vi "Vision Processing.vi"(8 "error in (no error)":errorcluster, 11 "Image Size":T2=enum."320x240") -> ()   [LabVIEW 2015]
uses:
  <vilib>/Rock Robotics/WPI/Camera/WPI_CameraImageSize.ctl
  SubSystems/Vision Support Code/Camera Types.ctl
  <vilib>/Rock Robotics/WPI/Camera/WPI_CameraFrameRate.ctl
  <vilib>/Rock Robotics/WPI/Camera/WPI_CameraWhite Balance Values.ctl
  <vilib>/Rock Robotics/WPI/Camera/WPI_CameraExposure Values.ctl
  Robot Global Data.vi
  <vilib>/vision/NI_Vision_Development_Module.lvlib
panel:
  in  "Frame Rate (fps)":T1=30 min=1 max=30
  in  "Image Size 2":T2=enum."320x240"
  in  "Goal Width":dbl=20.0
  in  "Center Right":dbl=170.0
  in  "Center Left":dbl=150.0
  in  "Maximum Shooting Distance":dbl
  in  "Distance Method":u16(ring)=2 items=["Default", "Center Calculations", "Hybrid", "Ratios"]
  in  "Camera Distance\nfrom Ground (in)":dbl
  out "More Detection":T3(array[cluster])
  in  "Mask Color":i32=1
  in  "Camera Type":T4=enum."MS HD3000 640x480"
  out "ms to process":u32
  in  "LED Color":T5={"Hue"={91.12518353230051, 179.40124989546868}, "Sat"={197.32142857142858, 255.0}, "Val"={182.14285714285714, 255.0}} {"Hue" scale=0.0..255.0 scale format="%#_3g"}
  out "Qualified Particles":i32
  in  "Aspect Fudge Factor":dbl=1.0
  in  "Min Score Threshold":i32=75
  out "Masked":T6(plugin-control)
  out "Original Image":T6(plugin-control)
  out "Sorted Particle Scores":T7(array[cluster]) {"Moment Factor" format="%#_3g"; "Aspect Ratio" format="%#_3g"; "Area to CH" format="%#_3g"; "X" format="%#_3g"; "Y" format="%#_3g"}
  out "Highest Avg Score":dbl
  out "Detected Targets":T8(array[cluster]) {"Normalized Rect"."Numeric 5" format="%#_2g"; "Normalized Rect"."Numeric 3" format="%#_2g"; "Normalized Rect"."Numeric 2" format="%#_2g"; "Normalized Rect"."Numeric" format="%#_2g"}
  out "fps":dbl
  # "Density Profile"
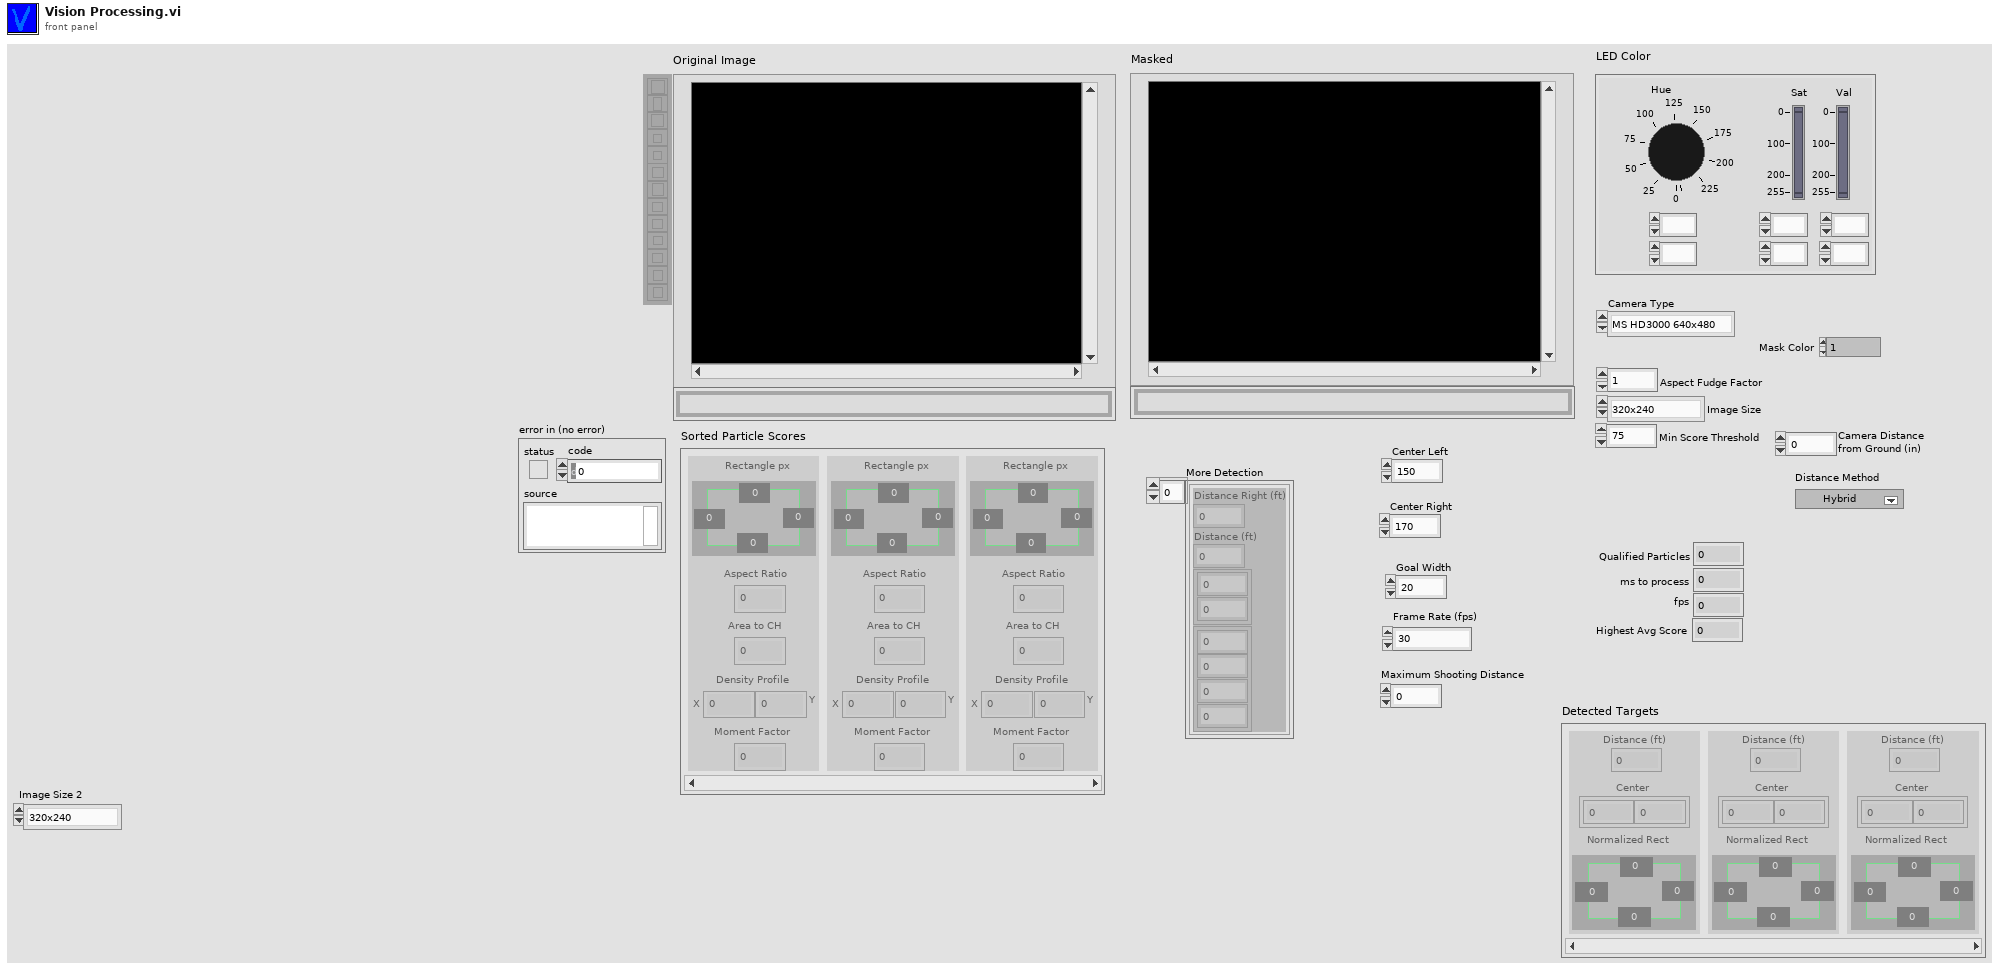
[diagram p1: front panel]
types:
  T1 = typedef "WPI_CameraFrameRate.ctl" = u32
  T2 = typedef "WPI_CameraImageSize.ctl" = enum16{"640x480", "320x240", "160x120", "Custom"}
  T3 = cluster{"Distance Right (ft)":dbl, "Distance (ft)":dbl, cluster{dbl, dbl}, cluster{dbl, dbl, dbl, dbl}}[]
  T4 = typedef "Camera Types.ctl" = enum16{"206", "1011", "1013", "MS HD3000 square", "MS HD3000 640x480"}
  T5 = cluster{"Hue":cluster{dbl, dbl}, "Sat":cluster{dbl, dbl}, "Val":cluster{dbl, dbl}}
  T6 = typedef "IMAQ Image.ctl" = refnum<image>
  T7 = cluster{"Rectangle px":cluster{"Numeric":dbl, "Numeric 2":dbl, "Numeric 3":dbl, "Numeric 5":dbl}, "Aspect Ratio":dbl, "Area to CH":dbl, "X":dbl, "Y":dbl, "Moment Factor":dbl}[]
  T8 = cluster{"Distance (ft)":dbl, "Center":cluster{dbl, dbl}, "Normalized Rect":cluster{"Numeric":dbl, "Numeric 2":dbl, "Numeric 3":dbl, "Numeric 5":dbl}}[]
  T9 = typedef "WPI_CameraExposure Values.ctl" = enum16{"Auto", "Flicker-free 50 Hz", "Flicker-free 60 Hz", "Hold current", "Custom"}
  T10 = typedef "WPI_CameraWhite Balance Values.ctl" = enum16{"Auto", "Fixed indoor", "Fixed outdoor 1", "Fixed outdoor 2", "Fixed fluorescent 1", "Fixed fluorescent 2", "Hold current", "Custom"}
  T11 = typedef "Image Type" = u32
  T12 = typedef "Particle Parameters" = i32
  T13 = typedef "WPI_CameraDevRef.ctl" = cluster{"Camera Address":string, "CameraStatus":errorcluster}
  T14 = cluster{"Bounding box":cluster{"left":dbl, "top":dbl, "right":dbl, "bottom":dbl}, "Aspect Ratio":dbl, "Area to CH":dbl, "X Mask":dbl, "Y Mask":dbl, "Moment":dbl}[]
  T15 = cluster{"Numeric":dbl, "Numeric":dbl, dbl, dbl, "Numeric":dbl, "Numeric":dbl}[]
  T16 = cluster{"Rectangle":cluster{"Numeric":dbl, "Numeric 2":dbl, "Numeric 3":dbl, "Numeric 5":dbl}, "L":dbl, "Area to CH":dbl, "X":dbl, "Y":dbl, "Moment Factor":dbl}[]
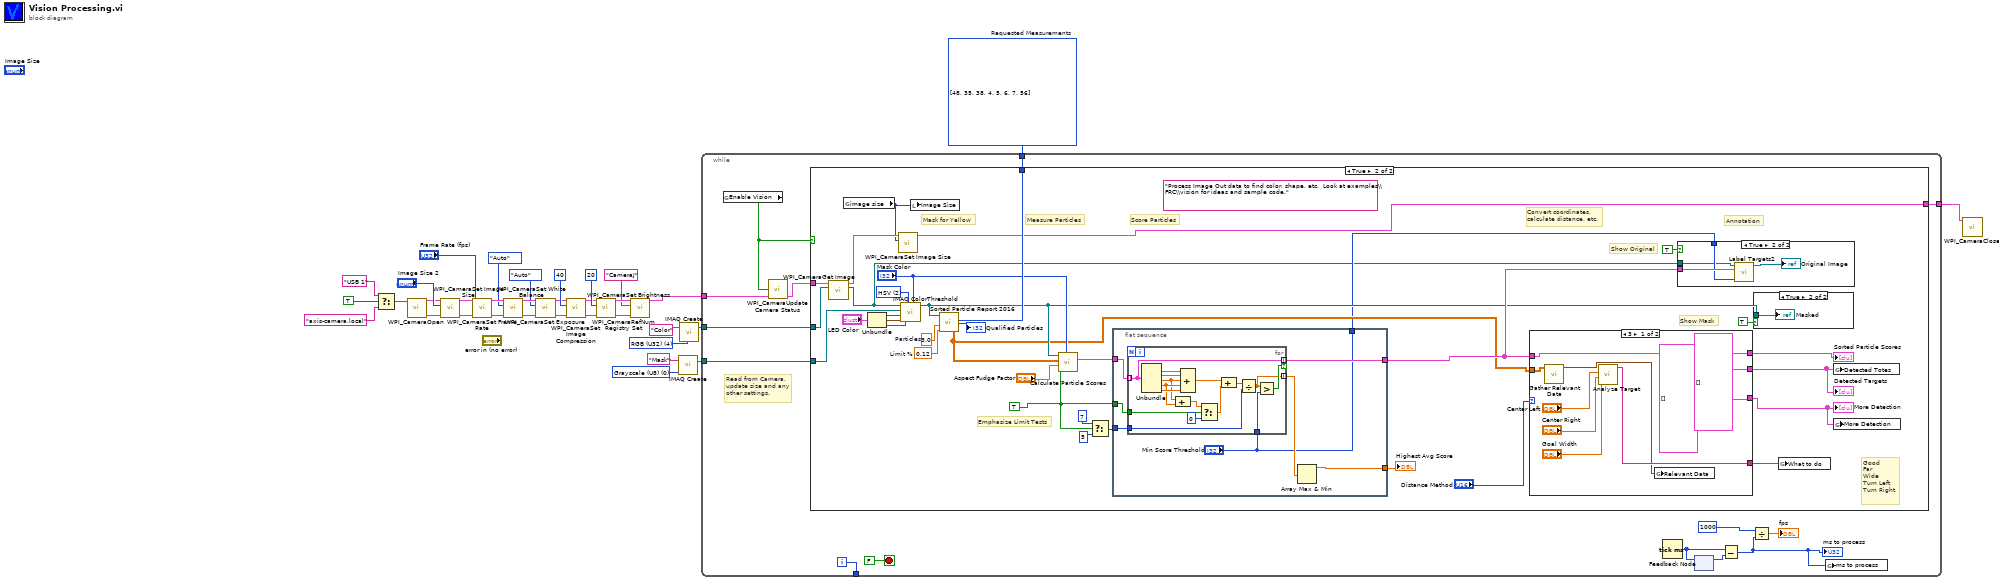
[diagram p0: block diagram]
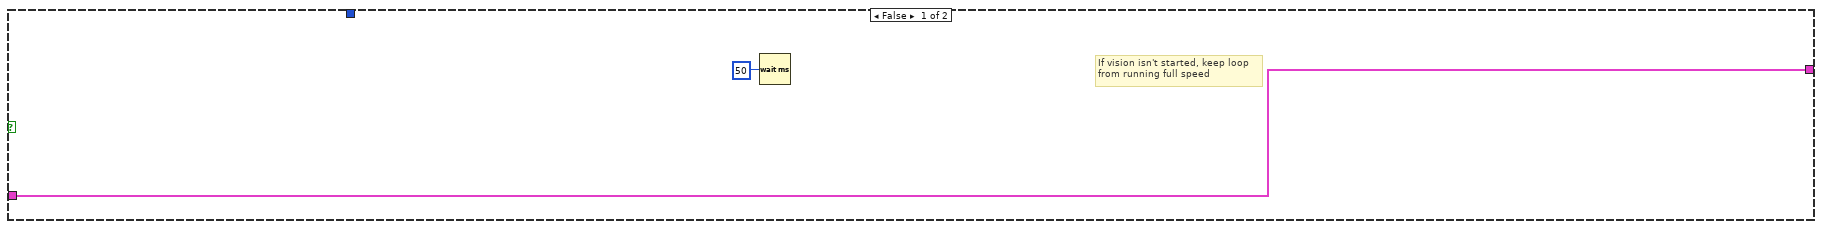
[diagram p2: hidden frame]
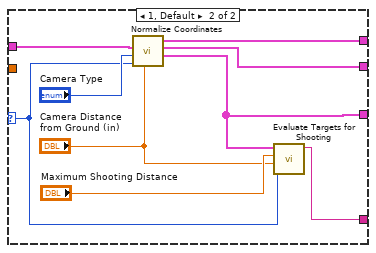
[diagram p3: hidden frame]
diagram:
  w30 = T11 4 items=["Grayscale (U8)", "Grayscale (I16)", "Grayscale (SGL)", "Complex (CSG)", "RGB (U32)", "HSL (U32)", "RGB (U64)", "Grayscale (U16)"] ("Image Type")
  w32 = T12[] [48, 35, 38, 4, 5, 6, 7, 56] items=["Center of Mass X", "Center of Mass Y", "First Pixel X", "First Pixel Y", "Bounding Rect Left", "Bounding Rect Top", "Bounding Rect Right", "Bounding Rect Bottom", "Max Feret Diameter Start X", "Max Feret Diameter Start Y", "Max Feret Diameter End X", "Max Feret Diameter End Y", "Max Horiz. Segment Length Left", "Max Horiz. Segment Length Right", "Max Horiz. Segment Length Row", "-", "Bounding Rect Width", "Bounding Rect Height", "Bounding Rect Diagonal", "Perimeter", "Convex Hull Perimeter", "Holes' Perimeter", "Max Feret Diameter", "Equivalent Ellipse Major Axis", "Equivalent Ellipse Minor Axis", "Equivalent Ellipse Minor Axis (Feret)", "Equivalent Rect Long Side", "Equivalent Rect Short Side", "Equivalent Rect Diagonal", "Equivalent Rect Short Side (Feret)", "Average Horiz. Segment Length", "Average Vert. Segment Length", "Hydraulic Radius", "Waddel Disk Diameter", "-", "Area", "Holes' Area", "Particle & Holes' Area", "Convex Hull Area", "Image Area", "-", "Number of Holes", "Number of Horiz. Segments", "Number of Vert. Segments", "-", "Orientation", "Max Feret Diameter Orientation", "-", "% Area/Image Area", "% Area/(Particle & Holes' Area)", "Ratio of Equivalent Ellipse Axes", "Ratio of Equivalent Rect Sides", "-", "Elongation Factor", "Compactness Factor", "Heywood Circularity Factor", "Type Factor", "-", "Sum X", "Sum Y", "Sum XX", "Sum XY", "Sum YY", "Sum XXX", "Sum XXY", "Sum XYY", "Sum YYY", "-", "Moment of Inertia XX", "Moment of Inertia XY", "Moment of Inertia YY", "Moment of Inertia XXX", "Moment of Inertia XXY", "Moment of Inertia XYY", "Moment of Inertia YYY", "Norm. Moment of Inertia XX", "Norm. Moment of Inertia XY", "Norm. Moment of Inertia YY", "Norm. Moment of Inertia XXX", "Norm. Moment of Inertia XXY", "Norm. Moment of Inertia XYY", "Norm. Moment of Inertia YYY", "Hu Moment 1", "Hu Moment 2", "Hu Moment 3", "Hu Moment 4", "Hu Moment 5", "Hu Moment 6", "Hu Moment 7"]  # Requested Measurements
  w34 = T11 0 items=["Grayscale (U8)", "Grayscale (I16)", "Grayscale (SGL)", "Complex (CSG)", "RGB (U32)", "HSL (U32)", "RGB (U64)", "Grayscale (U16)"] ("Image Type")
  n1 = Select(t="USB 1" ("format string"), s=TRUE ("dot notation? (F)"), f="axis-camera.local" ("format string")) -> (s? t:f=w4:string)
  n2 = call <vilib>:"WPI_CameraOpen.vi"("Camera Address"=w4) -> ("error out"=w15:errorcluster, "CameraDevRef"=w16:T13)  [unwired: 1 in, 8 out]
  n3 = call <vilib>:"WPI_CameraSet Image Size.vi"("error in (no error)"=w15, "Image Size"="Image Size 2", "CameraDevRef"=w16) -> ("error out"=w14:errorcluster, "CameraDevRef Out"=w17:T13)  [unwired: 1 in, 6 out]
  n4 = call <vilib>:"WPI_CameraSet Frame Rate.vi"("error in (no error)"=w14, "Frame Rate (fps)"="Frame Rate (fps)", "CameraDevRef"=w17) -> ("error out"=w13:errorcluster, "CameraDevRef Out"=w19:T13)  [unwired: 7 out]
  n5 = call <vilib>:"WPI_CameraSet White Balance.vi"("error in (no error)"=w13, "White Balance"=WPI_CameraWhite_Balance_Values."Auto", "CameraDevRef"=w19) -> ("error out"=w12:errorcluster, "CameraDevRef Out"=w18:T13)  [unwired: 1 in, 6 out]
  n6 = call <vilib>:"WPI_CameraSet Exposure.vi"("error in (no error)"=w12, "Exposure"=WPI_CameraExposure_Values."Auto", "CameraDevRef"=w18) -> ("error out"=w11:errorcluster, "CameraDevRef Out"=w21:T13)  [unwired: 1 in, 6 out]
  n7 = call <vilib>:"WPI_CameraSet Image Compression.vi"("error in (no error)"=w11, "Compression"=40, "CameraDevRef"=w21) -> ("error out"=w10:errorcluster, "CameraDevRef Out"=w20:T13)  [unwired: 7 out]
  n8 = call <vilib>:"WPI_CameraSet Brightness.vi"("error in (no error)"=w10, "Brightness"=20, "CameraDevRef"=w20) -> ("error out"=w9:errorcluster, "CameraDevRef Out"=w27:T13)  [unwired: 7 out]
  n9 = call <vilib>:"WPI_CameraRefNum Registry Set.vi"("error in (no error)"=w9, "refnum name"="CameraJ", "CameraDevRef"=w27) -> ("CameraDevRef"=w2:T13)  [unwired: 1 in, 7 out]
  n10 = call "IMAQ Create"("Image Name"="Mask", "Image Type"=w34) -> ("New Image"=w33:T6)  [unwired: 2 in, 2 out]
  n11 = call "IMAQ Create"("Image Name"="Color", "Image Type"=w30) -> ("New Image"=w29:T6)  [unwired: 3 in, 1 out]
  n12 = while {
    tunnel: w33 -> [w47]
    tunnel: w32 -> [w46]
    tunnel: [w43] -> _
    tunnel: w29 -> [w40]
    tunnel: w2 -> [w38]
    tunnel: [w36] -> w1
    i -> [w43]
    stop <- FALSE stop-if-true
    # "Read from Camera,\nupdate size and any\nother settings."
    n13 = global read "Robot Global Data.vi" "Enable Vision"() -> (w39:bool)
    n14 = call <vilib>:"WPI_CameraUpdate Camera Status.vi"("CameraDevRef In"=w38, "Enable Vision"=w39) -> ("CameraDevRef Out"=w37:T13)  [unwired: 3 in]
    n15 = case shown="True" w39 {
      tunnel: w47 -> [_ w85]
      tunnel: w46 -> [_ w74]
      tunnel: w40 -> [_ w58]
      tunnel: w37 -> [w49 w59]
      tunnel: [w49 w55] -> w36
      frame False {
        # "If vision isn't started, keep loop\nfrom running full speed"
        n16 = Wait (ms)(milliseconds to wait=u32 50) -> ()  [unwired: 1 out]
      }
      frame True {
        w63 = TRUE ("s")
        w80 = u16 2 items=["RGB", "HSL", "HSV", "HSI"] ("Color Mode")
        (unwired) "Process Image Out data to find color, shape, etc.  Look at examples\\FRC\\vision for ideas and sample code."
        w73 = 0.12  # Limit %
        w72 = 3.0  # Particles
        # "Show Mask"
        # "Show Original"
        # "Emphasize Limit Tests"
        # "Good\nFar\nWide\nTurn Left\nTurn Right"
        # "Measure Particles"
        # "Convert coordinates,\ncalculate distance, etc."
        # "Annotation"
        # "Score Particles"
        # "Mask for Yellow"
        n17 = call <vilib>:"WPI_CameraGet Image.vi"("Image"=w58, "CameraDevRef"=w59) -> ("Image Out"=w51:T6, "CameraDevRef Out"=w57:T13)  [unwired: 7 in, 1 out]
        n18 = global read "Robot Global Data.vi" "image size"() -> (w56:T2)
        n19 = Unbundle("LED Color") -> ("Hue"=w84:cluster{dbl, dbl}, "Sat"=w83:cluster{dbl, dbl}, "Val"=w82:cluster{dbl, dbl})
        n20 = call <vilib>:"WPI_CameraSet Image Size.vi"("Image Size"=w56, "CameraDevRef"=w57) -> ("CameraDevRef Out"=w55:T13)  [unwired: 2 in, 7 out]
        n21 = call "IMAQ ColorThreshold"("Blue or Luma or Val or Inten Range"=w82, "Replace Value"="Mask Color", "Green or Sat Range"=w83, "Color Mode"=w80, "Red or Hue Range"=w84, "Image Dst"=w85, "Image Src"=w51) -> ("Image Dst Out"=w67:T6)  [unwired: 3 in, 1 out]
        n22 = local write "Image Size"(w56) -> ()
        n23 = call "Sorted Particle Report 2016.vi"("Min Area Size %"=w73, "Particle Count Limit"=w72, "Pixel Measurements"=w74, "Image in"=w67) -> ("Sorted Data"=w64:dbl[][], "Particles"=→"Qualified Particles":i32)
        n24 = call "Calculate Particle Scores.vi"("Pixel Value"="Mask Color", "Limit Tests?"=w63, "Aspect Fudge Factor"="Aspect Fudge Factor", "Sorted Data"=w64, "Image in"=w67) -> ("Scores"=w71:T14)  [unwired: 6 in]
        n25 = Select(t=7, s=w63, f=5) -> (s? t:f=w77:i32)
        n26 = flat-sequence {
          tunnel: w71 -> [w114]
          tunnel: w77 -> [w112]
          tunnel: [w115] -> w76
          tunnel: [w110] -> w69
          tunnel: w63 -> [w113]
          tunnel: ["Min Score Threshold"] -> w60
          frame #0 {
            n27 = for {
              tunnel: w114 -> [w129] mode=indexing
              tunnel: [w129] -> w110 mode=indexing if=w128
              tunnel: [w127] -> w111 mode=indexing
              tunnel: w112 -> [w126]
              tunnel: "Min Score Threshold" -> [w125]
              tunnel: w113 -> [w118]
              n28 = Unbundle(w129) -> ("Aspect Ratio"=w131:dbl, "Area to CH"=w130:dbl, "X Mask"=w120:dbl, "Y Mask"=w121:dbl, "Moment"=w122:dbl)  [unwired: 1 out]
              n29 = Compound Arithmetic op=ADD(w120, w121) -> (w119:dbl)
              n30 = Compound Arithmetic op=ADD(w131, w130, w120, w121, w122) -> (w124:dbl)
              n31 = Select(t=w119, s=w118, f=0) -> (s? t:f=w117:dbl)
              n32 = Compound Arithmetic op=ADD(w124, w117) -> (w123:dbl)
              n33 = Divide(x=w123, y=w126) -> (x/y=w127:dbl)
              n34 = Greater?(x=w127, y=w125) -> (0:w128:bool)
            }
            n35 = Array Max & Min(array=w111) -> (max value=w115:dbl)  [unwired: 3 out]
          }
        }
        n36 = case shown="3" "Distance Method" {
          selector: "Distance Method" -> [_ w96]
          tunnel: w69 -> [w89 w103]
          tunnel: [w89 w102] -> w66
          tunnel: [T8 [] ("Found Targets") w101] -> w52
          tunnel: [T3 [] ("Array") w99] -> w53
          tunnel: w64 -> [w94 _]
          tunnel: [w93 w95] -> w54
          frame 3 {
            n37 = call "Gather Relevant Data.vi"("Sorted Data"=w94) -> ("Relevant Data"=w86:T15)  [unwired: 10 in]
            n38 = call "Analyze Target.vi"("Goal Width"="Goal Width", "Center Right"="Center Right", "Center Left"="Center Left") -> ("What to do"=w93:string)  [unwired: 8 in]
            n39 = global write "Robot Global Data.vi" "Relevant Data"(w86) -> ()
          }
          frame 1, Default {
            n40 = call "Normalize Coordinates.vi"("Camera Distance\nfrom Ground (in)"="Camera Distance\nfrom Ground (in)", "Distance Method"=w96, "Camera Type"="Camera Type", "Targets"=w103) -> ("Array"=w99:T3, "Found Targets"=w101:T8, "Sorted Scores"=w102:T16)  [unwired: 5 in]
            n41 = call "Evaluate Targets for Shooting.vi"("Distance Method"=w96, "Camera Distance\nfrom Ground (in)"="Camera Distance\nfrom Ground (in)", "Maximum Shooting Distance"="Maximum Shooting Distance", "More Detection"=w99) -> ("What to do"=w95:string)  [unwired: 6 in]
          }
        }
        "Sorted Particle Scores" <- w66
        "Detected Targets" <- w52
        "More Detection" <- w53
        n42 = case shown="True" TRUE {
          tunnel: w69 -> [_ w106]
          tunnel: w60 -> [_ w105]
          tunnel: w51 -> [_ w104]
          frame False {
          }
          frame True {
            n43 = call "Label Targets2.vi"("Score Threshold"=w105, "Targets"=w106, "Image in"=w104) -> ("Image out"=→"Original Image":T6)  [unwired: 8 in]
          }
        }
        n44 = case shown="True" TRUE {
          tunnel: w67 -> [_ w108]
          frame False {
          }
          frame True {
            "Masked" <- w108
          }
        }
        n45 = global write "Robot Global Data.vi" "What to do"(w54) -> ()
        n46 = global write "Robot Global Data.vi" "Detected Totes"(w52) -> ()
        n47 = global write "Robot Global Data.vi" "More Detection"(w53) -> ()
        "Highest Avg Score" <- w76
      }
    }
    n48 = Tick Count (ms)() -> (millisecond timer value=w44:u32)
    n49 = feedback-in #1(w44) -> ()
    n50 = feedback #1() -> (w45:u32)  [unwired: 1 in]
    n51 = Subtract(x=w44, y=w45) -> (x-y=w35:u32)
    "ms to process" <- w35
    n52 = Divide(x=1000 ("Brightness"), y=w35) -> (x/y=→"fps":dbl)
    n53 = global write "Robot Global Data.vi" "ms to process"(w35) -> ()
  }
  n54 = call <vilib>:"WPI_CameraClose.vi"("CameraDevRef"=w1) -> ()  [unwired: 1 in, 10 out]
